vi "Write Config Section.vi"(8 "error in":errorcluster, 11 "Data in":T1) -> (0 "error out":errorcluster, 3 "Data out":T1)   [LabVIEW 2021, in "Main INI.lvlib"]
uses:
  Main INI.lvlib
  <vilib>/Utility/config.llb/NI_LVConfig.lvlib
  <userlib>/_OpenG.lib/variantconfig/variantconfig.llb/openg_variant_configuration_file.lvlib
  Core Data.ctl
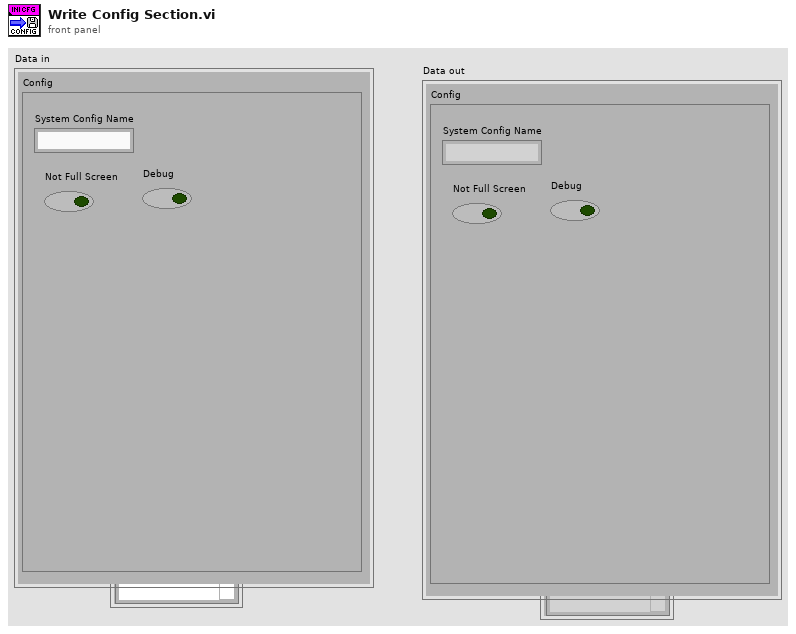
[diagram p1: front panel]
types:
  T1 = typedef "Main INI.lvlib/Core Data.ctl" = cluster{"Config":cluster{"System Config Name":string, "Not Full Screen":bool, "Debug":bool}}
  T2 = cluster{"System Config Name":string, "Not Full Screen":bool, "Debug":bool}
  T3 = typedef "NI_LVConfig.lvlib/Config Data RefNum.ctl" = refnum<k1>
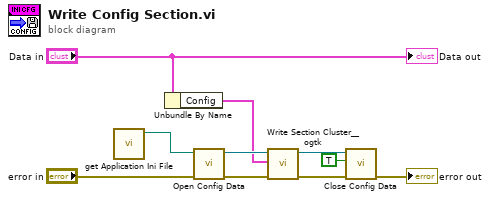
[diagram p0: block diagram]
diagram:
  n1 = call "get Application Ini File.vi"() -> ("Application Ini File"=w1:path)  [unwired: 11 in]
  n2 = Unbundle By Name("Data in") -> ("Config"=w3:T2)
  n3 = call <vilib>:"Open Config Data.vi"("error in (no error)"="error in", "configuration file path"=w1) -> ("error out"=w6:errorcluster, "refnum"=w7:T3)  [unwired: 7 in, 1 out]
  n4 = call <userlib>:"Write Section Cluster__ogtk.vi"("error in (no error)"=w6, "Section Formatted Cluster"=w3, "refnum"=w7) -> ("error out"=w8:errorcluster, "dup refnum"=w9:T3)  [unwired: 7 in]
  n5 = call <vilib>:"Close Config Data.vi"("error in (no error)"=w8, "write file if changed (T)"=TRUE, "refnum"=w9) -> ("error out"=→"error out":errorcluster)  [unwired: 7 in, 1 out]
  "Data out" <- "Data in"
